vi "Test Configuration - PAE.vi"(8 "error in":errorcluster, 11 "Test Configuration":T2={"Expected DUT Gain (dB)"=0.0, "Max Linear Range (dBm)"=0.0, "Compression Point (dB)"=0.0, "Pout at Pin (dBm)"=1.0, "RFSG Frequency Start (Hz)"=0.0, "RFSG Frequency Stop (Hz)"=0.0, "RFSG Number of Frequency Step"=0, "Power Start (dBm)"=0.0, "Power Stop(dBm)"=0.0, "Power Step Size (dB)"=0.0, "RBW (Hz)"=0.0, "Modes"={"RF Measurement Interval (s)"=0.001, "DC Measurement Interval (s)"=0.0, "Power Stimulus Mode"=enum."Constant Power and RF", "CP_CW_DC Source Delay (s)"=0.0002, "CP_PRF_RF Pulse Width (s)"=0.0009, "CP_PRF_PRI (s)"=0.015, "CP_PRF_DC Source Delay (s)"=0.0, "CP_PRF_RFmx Trigger Delay (s)"=0.2, "PP_PRF_RF Pulse Width (s)"=0.0, "PP_PRF_PRI (s)"=0.0, "PP_PRF_DC Pulse Width (s)"=0.0008, "PP_PRF_Bias Voltage Level (V)"=0.0, "PP_PRF_Bias Current Limit (A)"=0.2, "PP_PRF_DC Source Delay (s)"=0.0, "PP_PRF_RFmx Trigger Delay (s)"=0.0}} {"Pout at Pin (dBm)" format="%#pdBm"; "Modes"."PP_PRF_RFmx Trigger Delay (s)" format="%#ps"; "Modes"."PP_PRF_DC Source Delay (s)" format="%#ps"; "Modes"."PP_PRF_Bias Current Limit (A)" format="%#pA"; "Modes"."PP_PRF_Bias Voltage Level (V)" format="%#pV"; "Modes"."PP_PRF_DC Pulse Width (s)" format="%#ps"; "Modes"."PP_PRF_PRI (s)" format="%#ps"; "Modes"."PP_PRF_RF Pulse Width (s)" format="%#ps"; "Modes"."CP_PRF_RFmx Trigger Delay (s)" format="%#ps"; "Modes"."CP_PRF_DC Source Delay (s)" format="%#ps"; "Modes"."CP_PRF_PRI (s)" format="%#ps"; "Modes"."CP_PRF_RF Pulse Width (s)" format="%#ps"; "Modes"."CP_CW_DC Source Delay (s)" format="%#ps"; "Modes"."DC Measurement Interval (s)" format="%#_6p"; "RFSG Frequency Stop (Hz)" format="%#_6p"; "Power Start (dBm)" format="%#_6p"; "Power Stop(dBm)" format="%#_6p"; "RFSG Frequency Start (Hz)" format="%#_6p"; "Expected DUT Gain (dB)" step=1.0 format="%#_6p"}) -> (0 "error out":errorcluster, 2 "Compression Point (dB)":dbl, 3 "PAE Reference Out":T1)   [LabVIEW 2023]
uses:
  Controls/Test Config - Compression.ctl
  <vilib>/niPAEML/Typedefs/Session Handle.ctl
  <vilib>/niPAEML/PAE Reference.lvclass
  <vilib>/niPAEML/Configure RFSG Stimulus (CW).vi
  <vilib>/niPAEML/Configure DCPower Stimulus (Constant).vi
  <vilib>/niPAEML/Configure DCPower to RFSG Trigger (Automatic Routing).vi
  <vilib>/niPAEML/Configure RFSG Stimulus (Pulsed CW).vi
  <vilib>/niPAEML/Configure RFSG to RFmx Trigger (Automatic Routing) (Pulse).vi
  <vilib>/niPAEML/Configure RFmx to DCPower Trigger (Automatic Routing).vi
  <vilib>/niPAEML/Configure DCPower Stimulus (Pulsed).vi
  <vilib>/niPAEML/PAE Measurement.lvlib
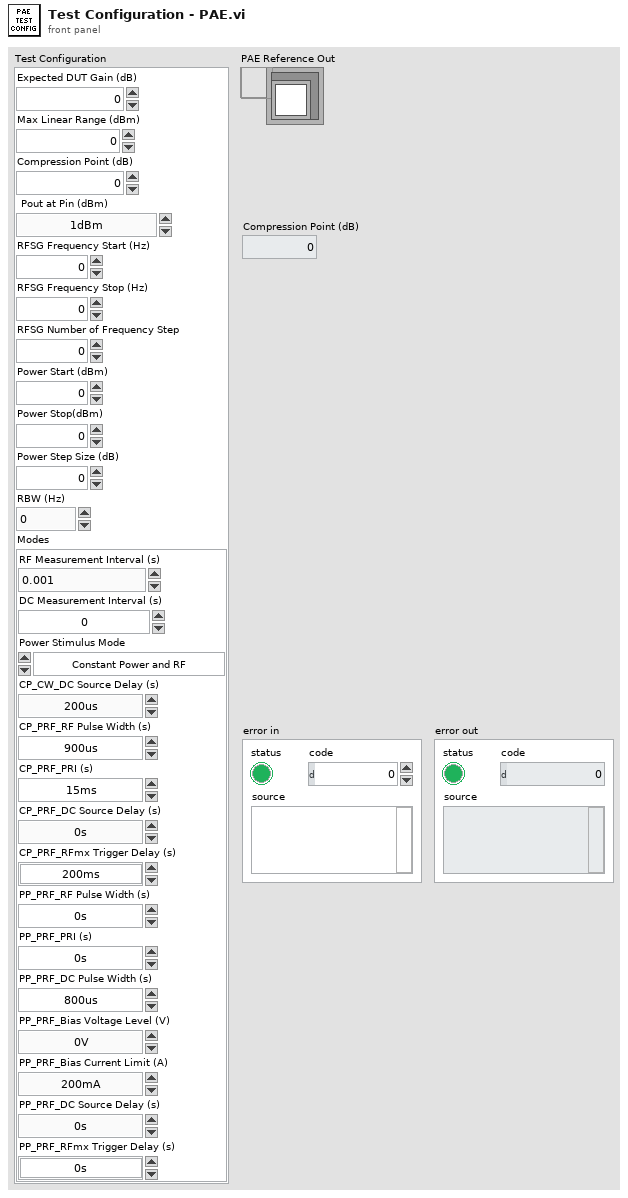
[diagram p1: front panel]
types:
  T1 = typedef "PAE Measurement.lvlib/PAE Reference.lvclass/Session Handle.ctl" = refnum<data-value>
  T2 = typedef "Test Config - Compression.ctl" = cluster{"Expected DUT Gain (dB)":dbl, "Max Linear Range (dBm)":dbl, "Compression Point (dB)":dbl, "Pout at Pin (dBm)":dbl, "RFSG Frequency Start (Hz)":dbl, "RFSG Frequency Stop (Hz)":dbl, "RFSG Number of Frequency Step":i32, "Power Start (dBm)":dbl, "Power Stop(dBm)":dbl, "Power Step Size (dB)":dbl, "RBW (Hz)":dbl, "Modes":cluster{"RF Measurement Interval (s)":dbl, "DC Measurement Interval (s)":dbl, "Power Stimulus Mode":enum16{"Constant Power and RF", "Constant Power and Pulsed RF", "Pulsed Power and RF"}, "CP_CW_DC Source Delay (s)":dbl, "CP_PRF_RF Pulse Width (s)":dbl, "CP_PRF_PRI (s)":dbl, "CP_PRF_DC Source Delay (s)":dbl, "CP_PRF_RFmx Trigger Delay (s)":dbl, "PP_PRF_RF Pulse Width (s)":dbl, "PP_PRF_PRI (s)":dbl, "PP_PRF_DC Pulse Width (s)":dbl, "PP_PRF_Bias Voltage Level (V)":dbl, "PP_PRF_Bias Current Limit (A)":dbl, "PP_PRF_DC Source Delay (s)":dbl, "PP_PRF_RFmx Trigger Delay (s)":dbl}}
  T3 = cluster{"RF Measurement Interval (s)":dbl, "DC Measurement Interval (s)":dbl, "Power Stimulus Mode":enum16{"Constant Power and RF", "Constant Power and Pulsed RF", "Pulsed Power and RF"}, "CP_CW_DC Source Delay (s)":dbl, "CP_PRF_RF Pulse Width (s)":dbl, "CP_PRF_PRI (s)":dbl, "CP_PRF_DC Source Delay (s)":dbl, "CP_PRF_RFmx Trigger Delay (s)":dbl, "PP_PRF_RF Pulse Width (s)":dbl, "PP_PRF_PRI (s)":dbl, "PP_PRF_DC Pulse Width (s)":dbl, "PP_PRF_Bias Voltage Level (V)":dbl, "PP_PRF_Bias Current Limit (A)":dbl, "PP_PRF_DC Source Delay (s)":dbl, "PP_PRF_RFmx Trigger Delay (s)":dbl}
  T4 = enum16{"Constant Power and RF", "Constant Power and Pulsed RF", "Pulsed Power and RF"}
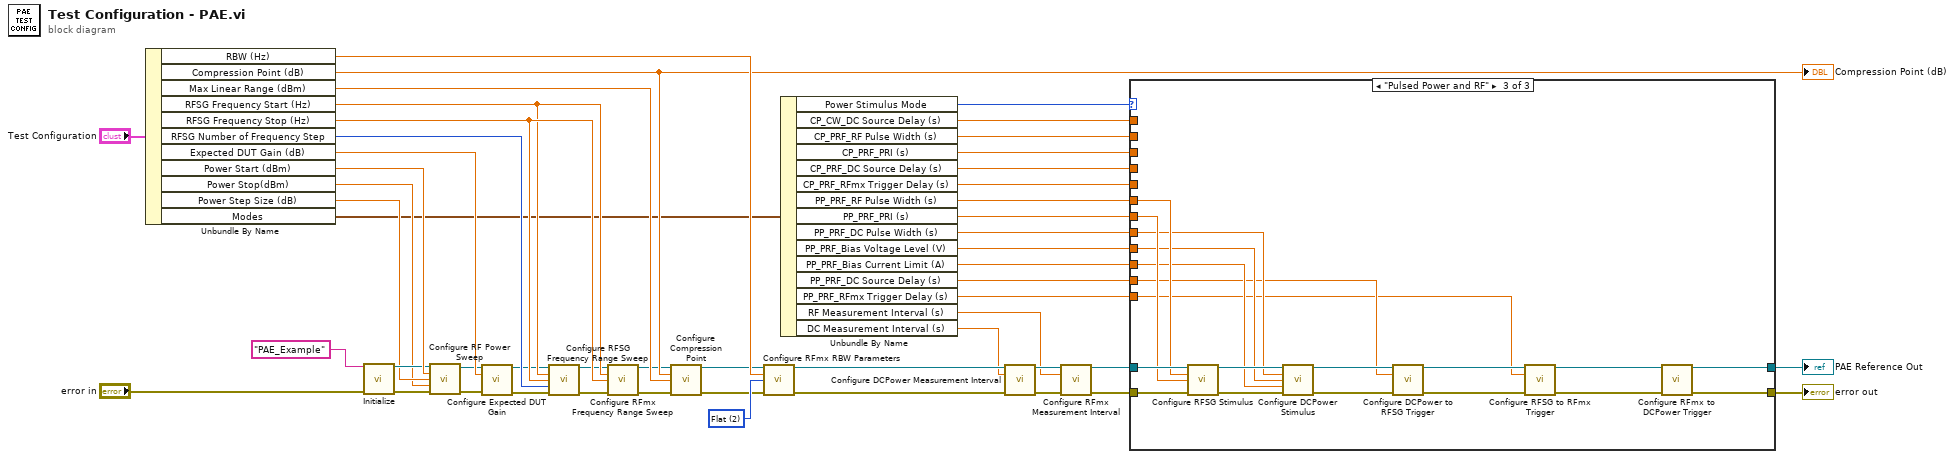
[diagram p0: block diagram]
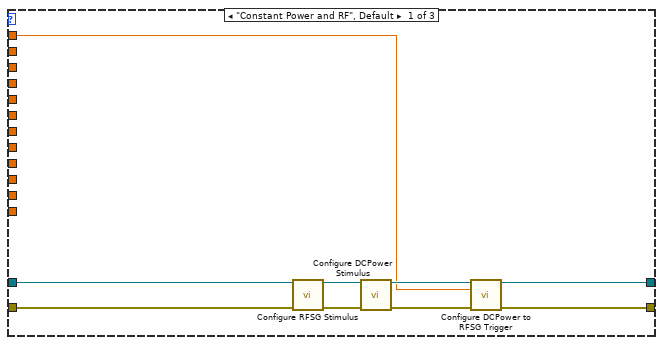
[diagram p2: hidden frame]
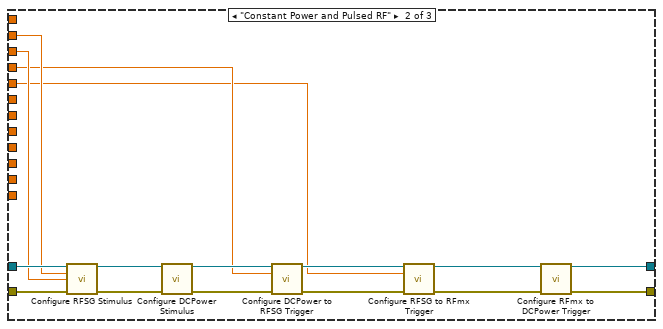
[diagram p3: hidden frame]
diagram:
  w38 = 2 items=["None"=5, "Gaussian"=1, "Flat"=2, "RRC"=6] ("RBW Filter Type")
  n1 = Unbundle By Name("Test Configuration") -> ("RBW (Hz)"=w48:dbl, "Compression Point (dB)"=w47:dbl, "Max Linear Range (dBm)"=w46:dbl, "RFSG Frequency Start (Hz)"=w45:dbl, "RFSG Frequency Stop (Hz)"=w50:dbl, "RFSG Number of Frequency Step"=w49:i32, "Expected DUT Gain (dB)"=w44:dbl, "Power Start (dBm)"=w43:dbl, "Power Stop(dBm)"=w25:dbl, "Power Step Size (dB)"=w26:dbl, "Modes"=w16:T3)
  "Compression Point (dB)" <- w47
  n2 = call <vilib>:"Initialize.vi"("Session Name"="PAE_Example", "error in"="error in") -> ("PAE Reference Out"=w27:T1, "error out"=w28:errorcluster)  [unwired: 12 in]
  n3 = call <vilib>:"Configure RF Power Sweep.vi"("PAE Reference In"=w27, "Initial Power (dBm)"=w43, "Power Step Size (dB)"=w26, "Final Power (dBm)"=w25, "error in"=w28) -> ("PAE Reference Out"=w35:T1, "error out"=w31:errorcluster)  [unwired: 9 in]
  n4 = call <vilib>:"Configure Expected DUT Gain.vi"("PAE Reference In"=w35, "Expected Gain (dB)"=w44, "error in"=w31) -> ("PAE Reference Out"=w36:T1, "error out"=w32:errorcluster)  [unwired: 11 in]
  n5 = call <vilib>:"Configure RFSG Frequency Range Sweep.vi"("PAE Reference In"=w36, "RFSG Start Frequency (Hz)"=w45, "RFSG Stop Frequency (Hz)"=w50, "Number of Frequency Steps"=w49, "error in"=w32) -> ("PAE Reference Out"=w41:T1, "error out"=w40:errorcluster)  [unwired: 9 in]
  n6 = call <vilib>:"Configure RFmx Frequency Range Sweep.vi"("PAE Reference In"=w41, "RFmx Start Frequency (Hz)"=w45, "RFmx Stop Frequency (Hz)"=w50, "error in"=w40) -> ("PAE Reference Out"=w34:T1, "error out"=w33:errorcluster)  [unwired: 10 in]
  n7 = call <vilib>:"Configure Compression Point.vi"("PAE Reference In"=w34, "Compression Point (dB)"=w47, "Maximum Linear Range (dBm)"=w46, "error in"=w33) -> ("PAE Reference Out"=w29:T1, "error out"=w30:errorcluster)  [unwired: 10 in]
  n8 = call <vilib>:"Configure RFmx RBW Parameters.vi"("PAE Reference In"=w29, "RBW (Hz)"=w48, "RBW Filter Type"=w38, "error in"=w30) -> ("PAE Reference Out"=w18:T1, "error out"=w17:errorcluster)  [unwired: 10 in]
  n9 = Unbundle By Name(w16) -> ("Power Stimulus Mode"=w13:T4, "CP_CW_DC Source Delay (s)"=w12:dbl, "CP_PRF_RF Pulse Width (s)"=w11:dbl, "CP_PRF_PRI (s)"=w10:dbl, "CP_PRF_DC Source Delay (s)"=w9:dbl, "CP_PRF_RFmx Trigger Delay (s)"=w8:dbl, "PP_PRF_RF Pulse Width (s)"=w7:dbl, "PP_PRF_PRI (s)"=w6:dbl, "PP_PRF_DC Pulse Width (s)"=w5:dbl, "PP_PRF_Bias Voltage Level (V)"=w4:dbl, "PP_PRF_Bias Current Limit (A)"=w3:dbl, "PP_PRF_DC Source Delay (s)"=w2:dbl, "PP_PRF_RFmx Trigger Delay (s)"=w1:dbl, "RF Measurement Interval (s)"=w15:dbl, "DC Measurement Interval (s)"=w14:dbl)
  n10 = call <vilib>:"Configure DCPower Measurement Interval.vi"("PAE Reference In"=w18, "DCPower Measurement Interval (s)"=w14, "error in"=w17) -> ("PAE Reference Out"=w24:T1, "error out"=w23:errorcluster)  [unwired: 11 in]
  n11 = call <vilib>:"Configure RFmx Measurement Interval.vi"("PAE Reference In"=w24, "RF Measurement Interval (s)"=w15, "error in"=w23) -> ("PAE Reference Out"=w22:T1, "error out"=w21:errorcluster)  [unwired: 11 in]
  n12 = case shown="\"Pulsed Power and RF\"" w13 {
    tunnel: w22 -> [w57 w67 w86]
    tunnel: w21 -> [w56 w66 w85]
    tunnel: [w53 w65 w84] -> w20
    tunnel: [w52 w64 w83] -> w19
    tunnel: w12 -> [w51 _ _]
    tunnel: w11 -> [_ w63 _]
    tunnel: w10 -> [_ w62 _]
    tunnel: w9 -> [_ w61 _]
    tunnel: w8 -> [_ w60 _]
    tunnel: w7 -> [_ _ w82]
    tunnel: w6 -> [_ _ w81]
    tunnel: w5 -> [_ _ w80]
    tunnel: w4 -> [_ _ w79]
    tunnel: w3 -> [_ _ w78]
    tunnel: w2 -> [_ _ w77]
    tunnel: w1 -> [_ _ w76]
    frame "Constant Power and RF", Default {
      n13 = call-poly <vilib>:"Configure RFSG Stimulus.vi"("PAE Reference In"=w57, "error in"=w56) -> ("PAE Reference Out"=w55:T1, "error out"=w54:errorcluster)  [unwired: 12 in]
      n14 = call-poly <vilib>:"Configure DCPower Stimulus.vi"("PAE Reference In"=w55, "error in"=w54) -> ("PAE Reference Out"=w59:T1, "error out"=w58:errorcluster)  [unwired: 12 in]
      n15 = call-poly <vilib>:"Configure DCPower to RFSG Trigger.vi"("PAE Reference In"=w59, "DCPower Source Delay (s)"=w51, "error in"=w58) -> ("PAE Reference Out"=w53:T1, "error out"=w52:errorcluster)  [unwired: 11 in]
    }
    frame "Constant Power and Pulsed RF" {
      n16 = call-poly <vilib>:"Configure RFSG Stimulus.vi"("PAE Reference In"=w67, "Pulse Width (s)"=w63, "PRI (s)"=w62, "error in"=w66) -> ("PAE Reference Out"=w69:T1, "error out"=w68:errorcluster)  [unwired: 10 in]
      n17 = call-poly <vilib>:"Configure DCPower Stimulus.vi"("PAE Reference In"=w69, "error in"=w68) -> ("PAE Reference Out"=w71:T1, "error out"=w70:errorcluster)  [unwired: 12 in]
      n18 = call-poly <vilib>:"Configure DCPower to RFSG Trigger.vi"("PAE Reference In"=w71, "DCPower Source Delay (s)"=w61, "error in"=w70) -> ("PAE Reference Out"=w72:T1, "error out"=w73:errorcluster)  [unwired: 11 in]
      n19 = call-poly <vilib>:"Configure RFSG to RFmx Trigger.vi"("PAE Reference In"=w72, "RFmx Trigger Delay (s)"=w60, "error in"=w73) -> ("PAE Reference Out"=w74:T1, "error out"=w75:errorcluster)  [unwired: 11 in]
      n20 = call-poly <vilib>:"Configure RFmx to DCPower Trigger.vi"("PAE Reference In"=w74, "error in"=w75) -> ("PAE Reference Out"=w65:T1, "error out"=w64:errorcluster)  [unwired: 12 in]
    }
    frame "Pulsed Power and RF" {
      n21 = call-poly <vilib>:"Configure RFSG Stimulus.vi"("PAE Reference In"=w86, "Pulse Width (s)"=w82, "PRI (s)"=w81, "error in"=w85) -> ("PAE Reference Out"=w88:T1, "error out"=w87:errorcluster)  [unwired: 10 in]
      n22 = call-poly <vilib>:"Configure DCPower Stimulus.vi"("PAE Reference In"=w88, "Pulse Width (s)"=w80, "Bias Voltage Level (V)"=w79, "Bias Current Limit (A)"=w78, "error in"=w87) -> ("PAE Reference Out"=w90:T1, "error out"=w89:errorcluster)  [unwired: 9 in]
      n23 = call-poly <vilib>:"Configure DCPower to RFSG Trigger.vi"("PAE Reference In"=w90, "DCPower Source Delay (s)"=w77, "error in"=w89) -> ("PAE Reference Out"=w91:T1, "error out"=w92:errorcluster)  [unwired: 11 in]
      n24 = call-poly <vilib>:"Configure RFSG to RFmx Trigger.vi"("PAE Reference In"=w91, "RFmx Trigger Delay (s)"=w76, "error in"=w92) -> ("PAE Reference Out"=w93:T1, "error out"=w94:errorcluster)  [unwired: 11 in]
      n25 = call-poly <vilib>:"Configure RFmx to DCPower Trigger.vi"("PAE Reference In"=w93, "error in"=w94) -> ("PAE Reference Out"=w84:T1, "error out"=w83:errorcluster)  [unwired: 12 in]
    }
  }
  "error out" <- w19
  "PAE Reference Out" <- w20
